vi "Calculate wheel velocity.vi"(9 "Speed":dbl(slide) scale=0.0..1000.0, 10 "Direction (radians)":dbl(slide) scale=0.0..6.283185307, 11 "Number of Wheels":u8) -> (2 "Wheel speeds":dbl[](array[numeric]))   [LabVIEW 2013]
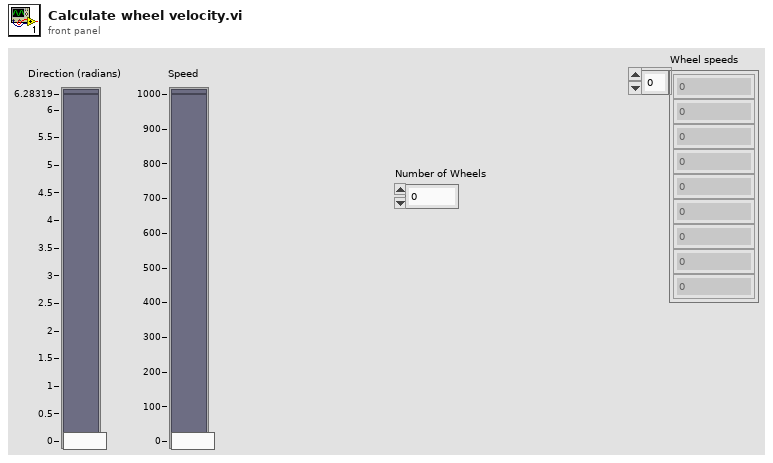
[diagram p1: front panel]
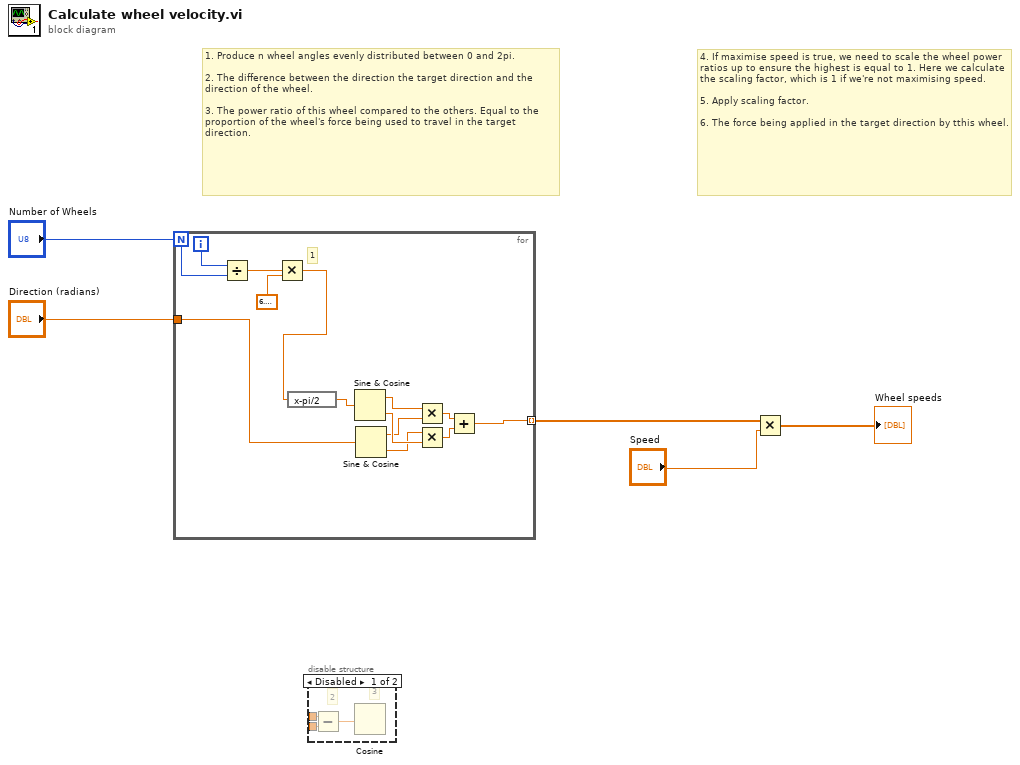
[diagram p0: block diagram]
diagram:
  # "4. If maximise speed is true, we need to scale the wheel power ratios up to ensure the highest is equal to 1. Here we calculate the scaling factor, which is 1 if we're not maximising speed.\n\n5. Apply scaling factor.\n\n6. The force being applied in the target direction by tthis wheel."
  # "1. Produce n wheel angles evenly distributed between 0 and 2pi.\n\n2. The difference between the direction the target direction and the direction of the wheel.\n\n3. The power ratio of this wheel compared to the others. Equal to the proportion of the wheel's force being used to travel in the target direction."
  n1 = for {
    N: "Number of Wheels" -> [w17]
    tunnel: "Direction (radians)" -> [w14]
    tunnel: [w6] -> w3 mode=indexing
    i -> [w16]
    # "1"
    n2 = Divide(x=w16, y=w17) -> (x/y=w19:dbl)
    n3 = Multiply(x=w19, y=6.283185307179586) -> (x*y=w15:dbl)
    n4 = expression code="x-pi/2"(w15) -> (w13:dbl)
    n5 = Sine & Cosine(0:w13) -> (1:w10:dbl, 2:w9:dbl)
    n6 = Sine & Cosine(0:w14) -> (1:w7:dbl, 2:w8:dbl)
    n7 = Multiply(x=w10, y=w7) -> (x*y=w12:dbl)
    n8 = Multiply(x=w8, y=w9) -> (x*y=w11:dbl)
    n9 = Add(x=w12, y=w11) -> (x+y=w6:dbl)
  }
  n10 = disable-structure shown="Disabled" {
    disable-tunnel: _ -> [w21 _]
    disable-tunnel: _ -> [w20 _]
    frame Disabled {
      # "3"
      # "2"
      n11 = Subtract(x=w20, y=w21) -> (x-y=w22:dbl)
      n12 = Cosine(x=w22) -> ()  [unwired: 1 out]
    }
    frame Enabled {
    }
  }
  n13 = Multiply(x=w3, y="Speed") -> (x*y=→"Wheel speeds":dbl[])
